vi "Init Bfr Rx - Create Buffer Options.vi"(8 "error in (no error)":errorcluster, 11 "Rx Loop Data in":T1 {"Buffer Resources"."Data Buffer" format="%016x"; "Buffer Option Support"."Ping Pong Buffer"."Active Buffer Ref" format="%016x"; "Buffer Option Support"."Cached Buffer"."Cache Buffer" format="%016x"}) -> (0 "error out":errorcluster, 3 "Rx Loop Data out":T1 {"Buffer Resources"."Data Buffer" format="%016x"; "Buffer Option Support"."Ping Pong Buffer"."Active Buffer Ref" format="%016x"; "Buffer Option Support"."Cached Buffer"."Cache Buffer" format="%016x"})   [LabVIEW 2019, in "UDP-Custom-Device Engine.lvlib"]
uses:
  UDP-Custom-Device Engine.lvlib
  Types/Engine - Buffered Rx Loop Data.ctl
  Types/Engine - General Resources.ctl
  <vilib>/NI VeriStand/VeriStand Data/Typedefs/Typedefs.Data Types.ctl
  Shared/Types/Shared - Duplex Settings.ctl
  Shared/Types/Shared - Header Details.ctl
  Types/Engine - Buffer Resources.ctl
  Shared/Types/Shared - Pointer Encoding.ctl
  Types/Engine - Rx Runtime Resources.ctl
  Types/Engine - Execution Config.ctl
  Shared/Types/Shared - Thread Management.ctl
  Types/Engine - Rx New Data Options Support.ctl
  Shared/Types/Shared - New Data Options.ctl
  Types/Engine - Buffered Rx Buffer Option Support.ctl
  Shared/Types/Shared - Receive Buffer Options.ctl
  Types/Engine - Buffered Rx Circular Buffer.ctl
  Types/Engine - Buffered Rx Cached Buffer.ctl
  Types/Engine - Buffered Rx Ping Pong Buffer.ctl
  Types/Engine - Buffered Rx Active Buffer.ctl
  Types/Engine - Buffered Rx Channel Refs.ctl
  <vilib>/NI/NIVS Inline Async API/_Data Access Engine/Data Access Engine/Types/Write.DVR.ctl
  <vilib>/NI/NIVS Inline Async API/_Data Access Engine/Access Type Classes/Write/Write.lvclass
  <vilib>/NI/NIVS Inline Async API/_Data Access Engine/Data Access Engine/Types/Read.DVR.ctl
  <vilib>/NI/NIVS Inline Async API/_Data Access Engine/Access Type Classes/Read/Read.lvclass
  Types/Engine - Buffered Rx Ping Pong Channels.ctl
  Types/Engine - Debug Resources.ctl
  <vilib>/NI/NIVS Inline Async API/_Data Access Engine/Access Type Classes/Write/Write.lvclass/Write.ctl
  <vilib>/NI VeriStand/VeriStand Data/Pointer Operations/Pointer.Write (1D U8).vi
  <vilib>/NI VeriStand/VeriStand Data/Pointer Operations/Pointer.Write (U8).vi
  <vilib>/NI VeriStand/VeriStand Data/Pointer Operations/Pointer.Write (U16).vi
  <vilib>/NI/NIVS Inline Async API/_Data Access Engine/Data Access Engine/Methods/Write.Data.vi
  <vilib>/NI/NIVS Inline Async API/_Data Access Engine/Access Type Classes/Write/Write.ProcessData.vi
  <vilib>/NI VeriStand/VeriStand Data/VeriStand Data.lvlib
  <vilib>/NI/NIVS Inline Async API/_Data Access Engine/Data Access Engine/Data Access Engine.lvclass
  Shared/UDP-Custom-Device Shared.lvlib
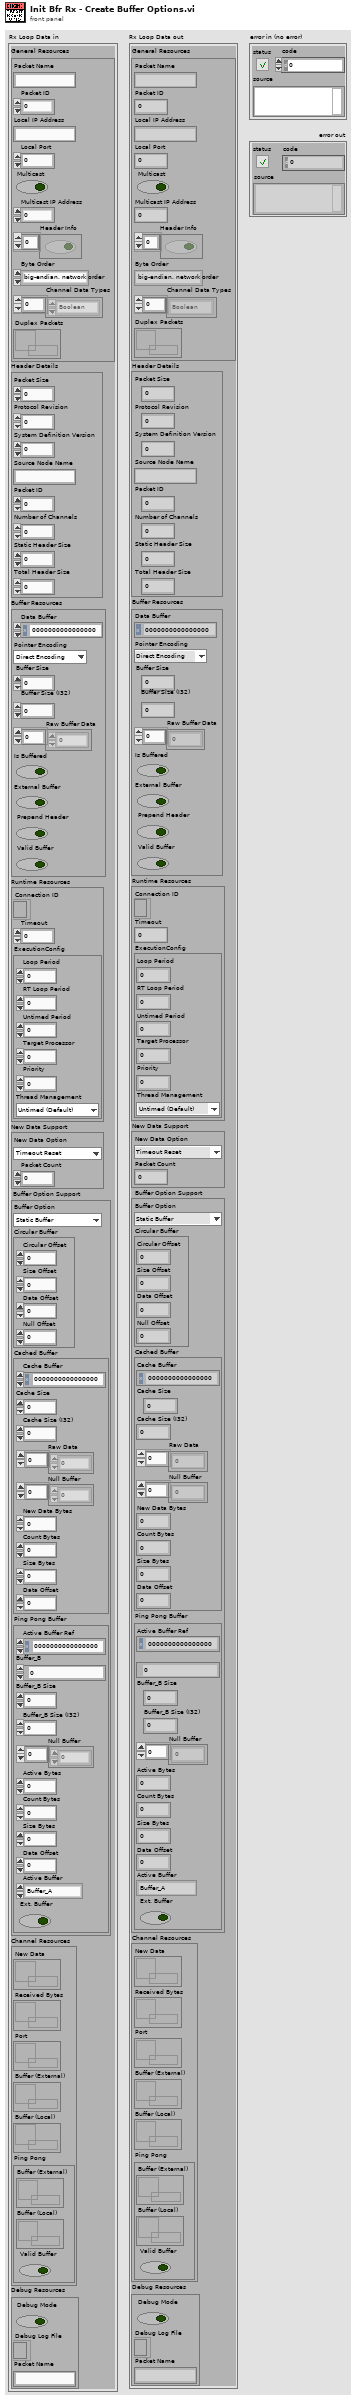
[diagram p1: front panel]
types:
  T1 = typedef "UDP-Custom-Device Engine.lvlib/Engine - Buffered Rx Loop Data.ctl" = cluster{"General Resources":T2, "Header Details":T4, "Buffer Resources":T5, "Runtime Resources":T7, "New Data Support":T10, "Buffer Option Support":T12, "Channel Resources":T18, "Debug Resources":T22}
  T2 = typedef "UDP-Custom-Device Engine.lvlib/Engine - General Resources.ctl" = cluster{"Packet Name":string, "Packet ID":i32, "Local IP Address":string, "Local Port":i32, "Multicast":bool, "Multicast IP Address":u32, "Header Info":bool[], "Byte Order":enum16{"big-endian, network order", "native, host order", "little-endian"}, "Channel Data Types":T3[], "Duplex Packets":refnum<data-value>}
  T3 = typedef "VeriStand Data.lvlib/Typedefs.Data Types.ctl" = enum16{"Boolean", "Single", "Double", "I8", "I16", "I32", "I64", "U8", "U16", "U32", "U64"}
  T4 = typedef "UDP-Custom-Device Shared.lvlib/Shared - Header Details.ctl" = cluster{"Packet Size":u16, "Protocol Revision":u8, "System Definition Version":u64, "Source Node Name":string, "Packet ID":u32, "Number of Channels":u32, "Static Header Size":u16, "Total Header Size":u16}
  T5 = typedef "UDP-Custom-Device Engine.lvlib/Engine - Buffer Resources.ctl" = cluster{"Data Buffer":u64, "Pointer Encoding":T6, "Buffer Size":u64, "Buffer Size (I32)":i32, "Raw Buffer Data":u8[], "Is Buffered":bool, "External Buffer":bool, "Prepend Header":bool, "Valid Buffer":bool}
  T6 = typedef "UDP-Custom-Device Shared.lvlib/Shared - Pointer Encoding.ctl" = enum16{"Direct Encoding", "Conversion Encoding"}
  T7 = typedef "UDP-Custom-Device Engine.lvlib/Engine - Rx Runtime Resources.ctl" = cluster{"Connection ID":refnum<k16>, "Timeout":i32, "ExecutionConfig":T8}
  T8 = typedef "UDP-Custom-Device Engine.lvlib/Engine - Execution Config.ctl" = cluster{"Loop Period":i64, "RT Loop Period":i64, "Untimed Period":u32, "Target Processor":i32, "Priority":i32, "Thread Management":T9}
  T9 = typedef "UDP-Custom-Device Shared.lvlib/Shared - Thread Management.ctl" = enum16{"Untimed (Default)", "Timed (High Priority)"}
  T10 = typedef "UDP-Custom-Device Engine.lvlib/Engine - Rx New Data Options Support.ctl" = cluster{"New Data Option":T11, "Packet Count":dbl}
  T11 = typedef "UDP-Custom-Device Shared.lvlib/Shared - New Data Options.ctl" = enum16{"Timeout Reset", "Counter"}
  T12 = typedef "UDP-Custom-Device Engine.lvlib/Engine - Buffered Rx Buffer Option Support.ctl" = cluster{"Buffer Option":T13, "Circular Buffer":T14, "Cached Buffer":T15, "Ping Pong Buffer":T16}
  T13 = typedef "UDP-Custom-Device Shared.lvlib/Shared - Receive Buffer Options.ctl" = enum16{"Static Buffer", "Circular Buffer", "Circular Buffer + Size", "Internal Cache", "Internal Cache + Size", "Ping Pong", "Ping Pong + Size"}
  T14 = typedef "UDP-Custom-Device Engine.lvlib/Engine - Buffered Rx Circular Buffer.ctl" = cluster{"Circular Offset":u64, "Size Offset":u64, "Data Offset":u64, "Null Offset":u64}
  T15 = typedef "UDP-Custom-Device Engine.lvlib/Engine - Buffered Rx Cached Buffer.ctl" = cluster{"Cache Buffer":u64, "Cache Size":u64, "Cache Size (I32)":i32, "Raw Data":u8[], "Null Buffer":u8[], "New Data Bytes":u64, "Count Bytes":u64, "Size Bytes":u64, "Data Offset":u64}
  T16 = typedef "UDP-Custom-Device Engine.lvlib/Engine - Buffered Rx Ping Pong Buffer.ctl" = cluster{"Active Buffer Ref":u64, "Buffer_B":u64, "Buffer_B Size":u64, "Buffer_B Size (I32)":i32, "Null Buffer":u8[], "Active Bytes":u64, "Count Bytes":u64, "Size Bytes":u64, "Data Offset":u64, "Active Buffer":T17, "Ext. Buffer":bool}
  T17 = typedef "UDP-Custom-Device Engine.lvlib/Engine - Buffered Rx Active Buffer.ctl" = enum16{"Buffer_A", "Buffer_B"}
  T18 = typedef "UDP-Custom-Device Engine.lvlib/Engine - Buffered Rx Channel Refs.ctl" = cluster{"New Data":T19, "Received Bytes":T19, "Port":T19, "Buffer (External)":T20, "Buffer (Local)":T19, "Ping Pong":T21}
  T19 = typedef "Data Access Engine.lvlib/Data Access Engine.lvclass/Write.DVR.ctl" = refnum<data-value>
  T20 = typedef "Data Access Engine.lvlib/Data Access Engine.lvclass/Read.DVR.ctl" = refnum<data-value>
  T21 = typedef "UDP-Custom-Device Engine.lvlib/Engine - Buffered Rx Ping Pong Channels.ctl" = cluster{"Buffer (External)":T20, "Buffer (Local)":T19, "Valid Buffer":bool}
  T22 = typedef "UDP-Custom-Device Engine.lvlib/Engine - Debug Resources.ctl" = cluster{"Debug Mode":bool, "Debug Log File":refnum<file>, "Packet Name":string}
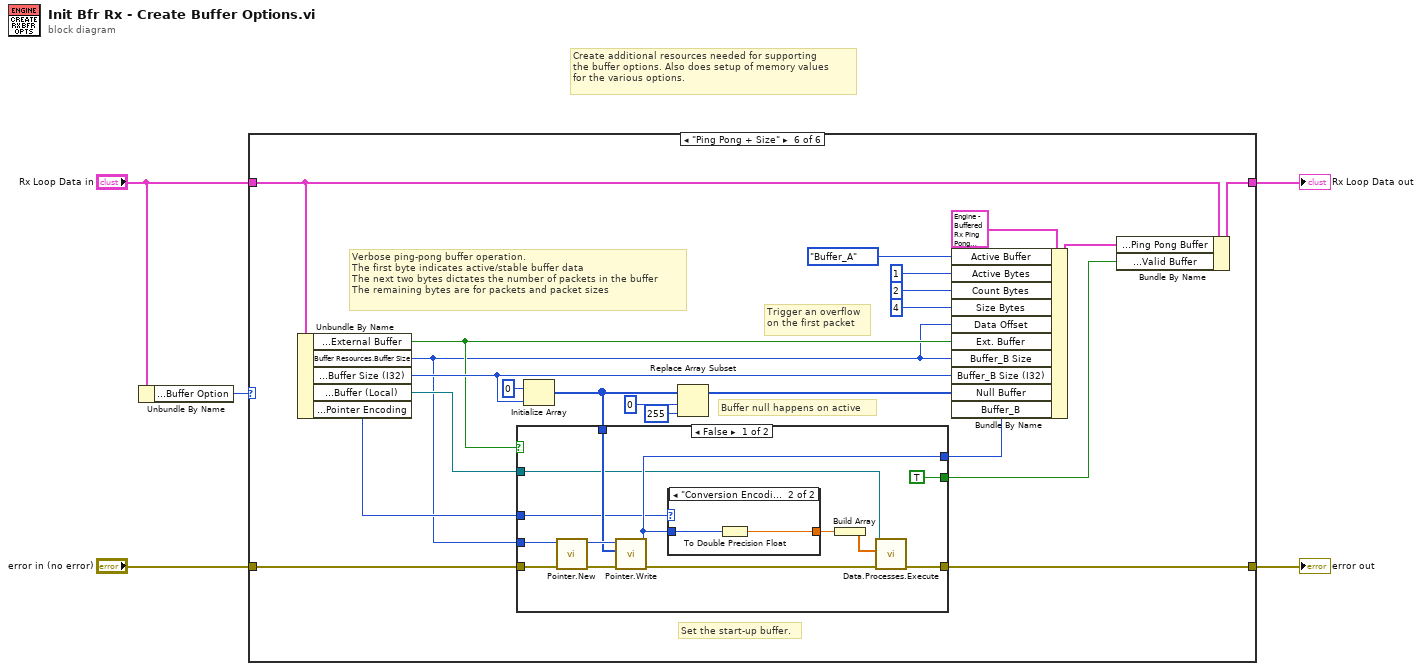
[diagram p0: block diagram]
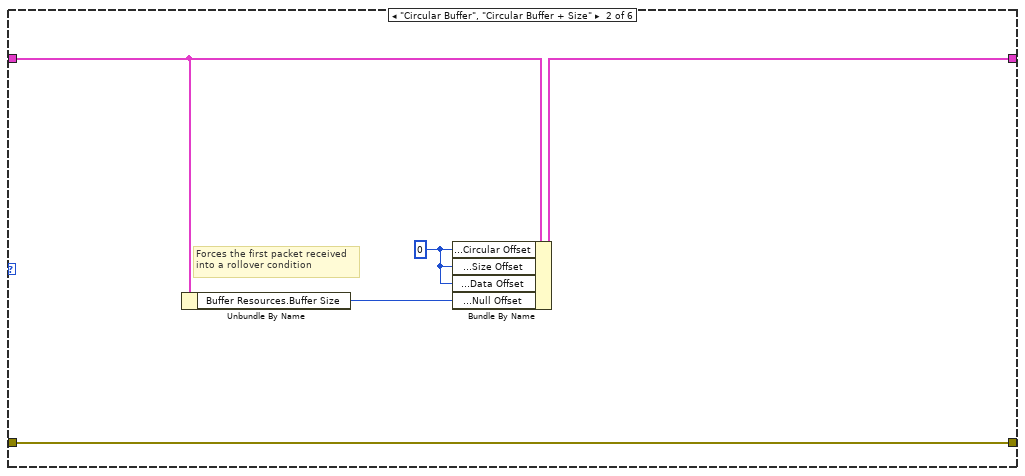
[diagram p3: hidden frame]
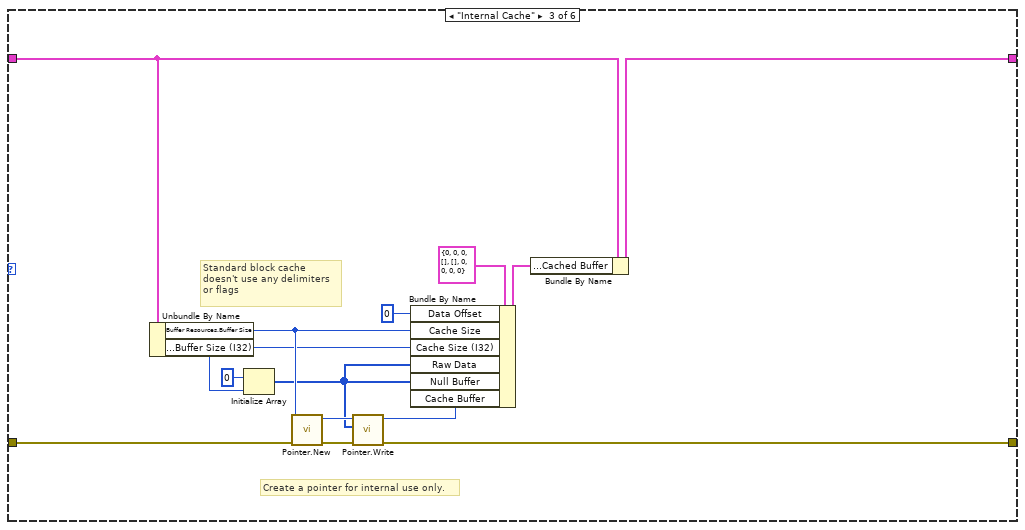
[diagram p4: hidden frame]
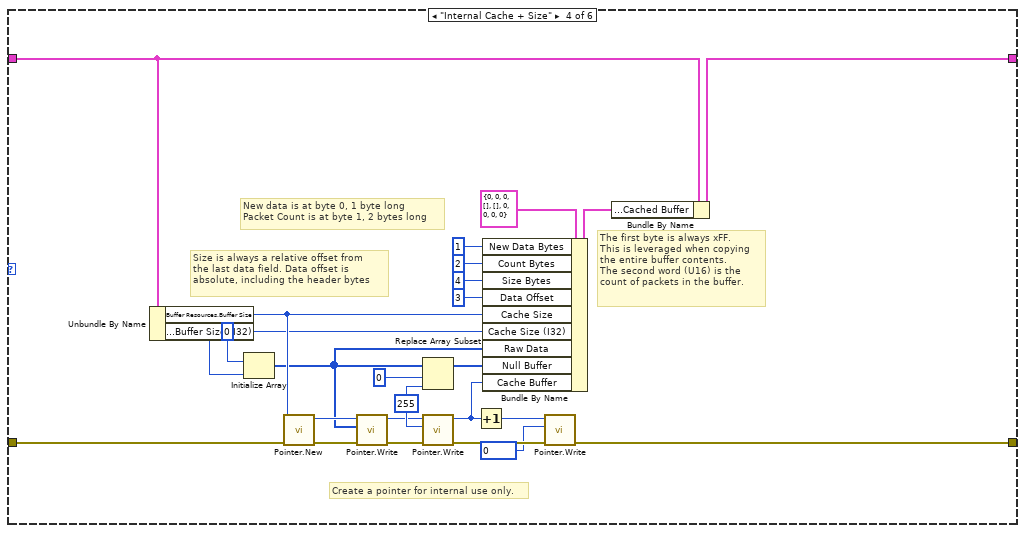
[diagram p5: hidden frame]
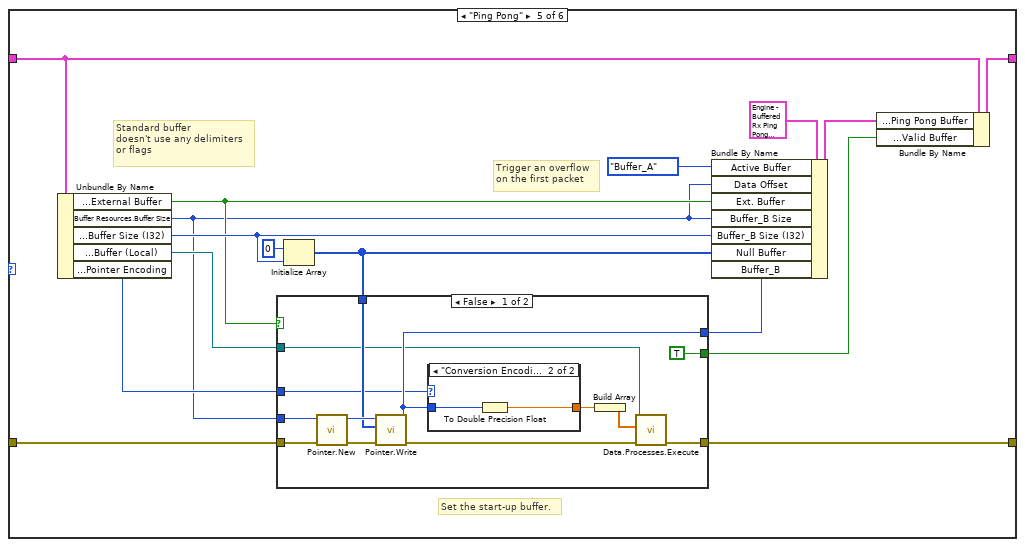
[diagram p6: hidden frame]
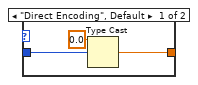
[diagram p7: hidden frame]
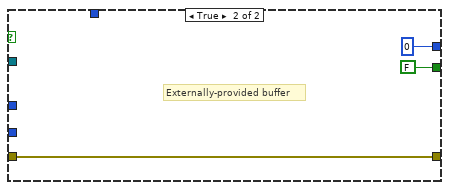
[diagram p8: hidden frame]
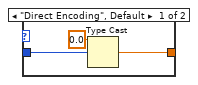
[diagram p9: hidden frame]
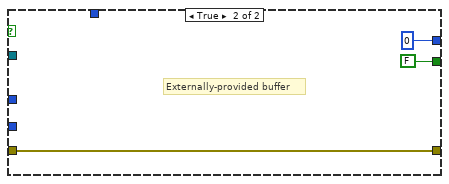
[diagram p10: hidden frame]
diagram:
  # "Create additional resources needed for supporting\nthe buffer options. Also does setup of memory values\nfor the various options."
  n1 = Unbundle By Name("Rx Loop Data in") -> ("Buffer Option Support.Buffer Option"=w1:T13)
  n2 = case shown="\"Ping Pong + Size\"" w1 {
    tunnel: [w7 w11 w26 w51 w67 w110] -> w5
    tunnel: "Rx Loop Data in" -> [w7 w10 w23 w48 w64 w107]
    tunnel: [w6 w12 w15 w38 w60 w103] -> w3
    tunnel: "error in (no error)" -> [w6 w12 w21 w45 w61 w104]
    frame Default {
    }
    frame "Circular Buffer", "Circular Buffer + Size" {
      w9 = u64 0 ("Buffer Option Support.Circular Buffer.Circular Offset")
      # "Forces the first packet received\ninto a rollover condition"
      n3 = Unbundle By Name(w10) -> ("Buffer Resources.Buffer Size"=w8:u64)
      n4 = Bundle By Name(cluster=w10, "Buffer Option Support.Circular Buffer.Circular Offset"=w9, "Buffer Option Support.Circular Buffer.Size Offset"=w9, "Buffer Option Support.Circular Buffer.Data Offset"=w9, "Buffer Option Support.Circular Buffer.Null Offset"=w8) -> (w11:T1)
    }
    frame "Internal Cache" {
      # "Standard block cache\ndoesn't use any delimiters\nor flags"
      # "Create a pointer for internal use only."
      n5 = Unbundle By Name(w23) -> ("Buffer Resources.Buffer Size"=w22:u64, "Buffer Resources.Buffer Size (I32)"=w20:i32)
      n6 = Initialize Array(u8 0 ("element"), w20) -> (w13:u8[])
      n7 = call <vilib>:"Pointer.New.vi"("error in (no error)"=w21, "size in bytes"=w22) -> ("error out"=w16:errorcluster, "pointer"=w18:u64)  [unwired: 8 in]
      n8 = call-poly <vilib>:"Pointer.Write.vi"("error in (no error)"=w16, "values"=w13, "pointer in"=w18) -> ("error out"=w15:errorcluster, "pointer out"=w17:u64)  [unwired: 6 in, 1 out]
      n9 = Bundle By Name(cluster=T15 {"Cache Buffer"=0, "Cache Size"=0, "Cache Size (I32)"=0, "Raw Data"=[], "Null Buffer"=[], "New Data Bytes"=0, "Count Bytes"=0, "Size Bytes"=0, "Data Offset"=0} ("Buffer Option Support.Cached Buffer"), "Data Offset"=u64 0 ("Buffer Option Support.Circular Buffer.Circular Offset"), "Cache Size"=w22, "Cache Size (I32)"=w20, "Raw Data"=w13, "Null Buffer"=w13, "Cache Buffer"=w17) -> (w24:T15)
      n10 = Bundle By Name(cluster=w23, "Buffer Option Support.Cached Buffer"=w24) -> (w26:T1)
    }
    frame "Internal Cache + Size" {
      w33 = u8 255 ("value")
      # "Size is always a relative offset from\nthe last data field. Data offset is\nabsolute, including the header bytes"
      # "The first byte is always xFF.\nThis is leveraged when copying\nthe entire buffer contents.\nThe second word (U16) is the\ncount of packets in the buffer."
      # "New data is at byte 0, 1 byte long\nPacket Count is at byte 1, 2 bytes long"
      # "Create a pointer for internal use only."
      n11 = Unbundle By Name(w48) -> ("Buffer Resources.Buffer Size"=w46:u64, "Buffer Resources.Buffer Size (I32)"=w44:i32)
      n12 = Initialize Array(u8 0 ("element"), w44) -> (w27:u8[])
      n13 = call <vilib>:"Pointer.New.vi"("error in (no error)"=w45, "size in bytes"=w46) -> ("error out"=w29:errorcluster, "pointer"=w31:u64)  [unwired: 8 in]
      n14 = call-poly <vilib>:"Pointer.Write.vi"("error in (no error)"=w29, "values"=w27, "pointer in"=w31) -> ("error out"=w28:errorcluster, "pointer out"=w30:u64)  [unwired: 6 in, 1 out]
      n15 = Replace Array Subset(array=w27, new element=w33, index=0) -> (w34:u8[])
      n16 = call-poly <vilib>:"Pointer.Write.vi"("error in (no error)"=w28, "value"=w33, "pointer in"=w30) -> ("error out"=w39:errorcluster, "pointer out"=w41:u64)  [unwired: 6 in, 1 out]
      n17 = Increment(x=w41) -> (x+1=w40:u64)
      n18 = Bundle By Name(cluster=T15 {"Cache Buffer"=0, "Cache Size"=0, "Cache Size (I32)"=0, "Raw Data"=[], "Null Buffer"=[], "New Data Bytes"=0, "Count Bytes"=0, "Size Bytes"=0, "Data Offset"=0} ("Buffer Option Support.Cached Buffer"), "New Data Bytes"=u64 1 ("Buffer Option Support.Circular Buffer.Circular Offset"), "Count Bytes"=u64 2 ("New Data Offset"), "Size Bytes"=u64 4 ("Buffer Option Support.Circular Buffer.Circular Offset"), "Data Offset"=u64 3, "Cache Size"=w46, "Cache Size (I32)"=w44, "Raw Data"=w27, "Null Buffer"=w34, "Cache Buffer"=w41) -> (w49:T15)
      n19 = call-poly <vilib>:"Pointer.Write.vi"("error in (no error)"=w39, "value"=u16 0, "pointer in"=w40) -> ("error out"=w38:errorcluster)  [unwired: 6 in, 2 out]
      n20 = Bundle By Name(cluster=w48, "Buffer Option Support.Cached Buffer"=w49) -> (w51:T1)
    }
    frame "Ping Pong" {
      # "Trigger an overflow\non the first packet"
      # "Set the start-up buffer."
      # "Standard buffer\ndoesn't use any delimiters\nor flags"
      n21 = Unbundle By Name(w64) -> ("Buffer Resources.External Buffer"=w59:bool, "Buffer Resources.Buffer Size"=w53:u64, "Buffer Resources.Buffer Size (I32)"=w66:i32, "Channel Resources.Ping Pong.Buffer (Local)"=w56:T19, "Buffer Resources.Pointer Encoding"=w57:T6)
      n22 = Initialize Array(u8 0 ("element"), w66) -> (w52:u8[])
      n23 = case shown="False" w59 {
        tunnel: w53 -> [w78 _]
        tunnel: w61 -> [w77 w88]
        tunnel: [w71 w88] -> w60
        tunnel: w52 -> [w76 _]
        tunnel: [w75 u64 0 ("pointer out")] -> w58
        tunnel: w57 -> [w74 _]
        tunnel: w56 -> [w70 _]
        tunnel: [TRUE FALSE] -> w55
        frame False {
          n24 = call <vilib>:"Pointer.New.vi"("error in (no error)"=w77, "size in bytes"=w78) -> ("error out"=w80:errorcluster, "pointer"=w79:u64)  [unwired: 8 in]
          n25 = call-poly <vilib>:"Pointer.Write.vi"("error in (no error)"=w80, "values"=w76, "pointer in"=w79) -> ("error out"=w72:errorcluster, "pointer out"=w75:u64)  [unwired: 6 in, 1 out]
          n26 = case shown="\"Conversion Encoding\"" w74 {
            tunnel: w75 -> [w83 w85]
            tunnel: [w82 w84] -> w73
            frame "Direct Encoding", Default {
              n27 = Type Cast(type=0.0, x=w83) -> (*(type *) &x=w82:dbl)
            }
            frame "Conversion Encoding" {
              n28 = To Double Precision Float(number=w85) -> (double precision float=w84:dbl)
            }
          }
          n29 = Build Array(w73) -> (w69:dbl[])
          n30 = call-poly <vilib>:"Data.Processes.Execute.vi"("error in (no error)"=w72, "Values"=w69, "Ref"=w70) -> ("error out"=w71:errorcluster)  [unwired: 8 in]
        }
        frame True {
          # "Externally-provided buffer"
        }
      }
      n31 = Bundle By Name(cluster=T16 {"Active Buffer Ref"=0, "Buffer_B"=0, "Buffer_B Size"=0, "Buffer_B Size (I32)"=0, "Null Buffer"=[], "Active Bytes"=0, "Count Bytes"=0, "Size Bytes"=0, "Data Offset"=0, "Active Buffer"=enum."Buffer_A", "Ext. Buffer"=FALSE} ("Ping Pong Buffer"), "Active Buffer"=Engine_-_Buffered_Rx_Active_Buffer."Buffer_A", "Data Offset"=w53, "Ext. Buffer"=w59, "Buffer_B Size"=w53, "Buffer_B Size (I32)"=w66, "Null Buffer"=w52, "Buffer_B"=w58) -> (w62:T16)
      n32 = Bundle By Name(cluster=w64, "Buffer Option Support.Ping Pong Buffer"=w62, "Channel Resources.Ping Pong.Valid Buffer"=w55) -> (w67:T1)
    }
    frame "Ping Pong + Size" {
      # "Buffer null happens on active"
      # "Trigger an overflow\non the first packet"
      # "Verbose ping-pong buffer operation.\nThe first byte indicates active/stable buffer data\nThe next two bytes dictates the number of packets in the buffer\nThe remaining bytes are for packets and packet sizes"
      # "Set the start-up buffer."
      n33 = Unbundle By Name(w107) -> ("Buffer Resources.External Buffer"=w102:bool, "Buffer Resources.Buffer Size"=w93:u64, "Buffer Resources.Buffer Size (I32)"=w109:i32, "Channel Resources.Ping Pong.Buffer (Local)"=w99:T19, "Buffer Resources.Pointer Encoding"=w100:T6)
      n34 = Initialize Array(u8 0 ("element"), w109) -> (w90:u8[])
      n35 = case shown="False" w102 {
        tunnel: w93 -> [w121 _]
        tunnel: w104 -> [w120 w131]
        tunnel: [w114 w131] -> w103
        tunnel: w90 -> [w119 _]
        tunnel: [w118 u64 0 ("pointer out")] -> w101
        tunnel: w100 -> [w117 _]
        tunnel: w99 -> [w113 _]
        tunnel: [TRUE FALSE] -> w98
        frame False {
          n36 = call <vilib>:"Pointer.New.vi"("error in (no error)"=w120, "size in bytes"=w121) -> ("error out"=w123:errorcluster, "pointer"=w122:u64)  [unwired: 8 in]
          n37 = call-poly <vilib>:"Pointer.Write.vi"("error in (no error)"=w123, "values"=w119, "pointer in"=w122) -> ("error out"=w115:errorcluster, "pointer out"=w118:u64)  [unwired: 6 in, 1 out]
          n38 = case shown="\"Conversion Encoding\"" w117 {
            tunnel: w118 -> [w126 w128]
            tunnel: [w125 w127] -> w116
            frame "Direct Encoding", Default {
              n39 = Type Cast(type=0.0, x=w126) -> (*(type *) &x=w125:dbl)
            }
            frame "Conversion Encoding" {
              n40 = To Double Precision Float(number=w128) -> (double precision float=w127:dbl)
            }
          }
          n41 = Build Array(w116) -> (w112:dbl[])
          n42 = call-poly <vilib>:"Data.Processes.Execute.vi"("error in (no error)"=w115, "Values"=w112, "Ref"=w113) -> ("error out"=w114:errorcluster)  [unwired: 8 in]
        }
        frame True {
          # "Externally-provided buffer"
        }
      }
      n43 = Replace Array Subset(array=w90, new element=u8 255 ("new element/subarray"), index=0) -> (w89:u8[])
      n44 = Bundle By Name(cluster=T16 {"Active Buffer Ref"=0, "Buffer_B"=0, "Buffer_B Size"=0, "Buffer_B Size (I32)"=0, "Null Buffer"=[], "Active Bytes"=0, "Count Bytes"=0, "Size Bytes"=0, "Data Offset"=0, "Active Buffer"=enum."Buffer_A", "Ext. Buffer"=FALSE} ("Ping Pong Buffer"), "Active Buffer"=Engine_-_Buffered_Rx_Active_Buffer."Buffer_A", "Active Bytes"=u64 1 ("New Data Bytes"), "Count Bytes"=u64 2, "Size Bytes"=u64 4, "Data Offset"=w93, "Ext. Buffer"=w102, "Buffer_B Size"=w93, "Buffer_B Size (I32)"=w109, "Null Buffer"=w89, "Buffer_B"=w101) -> (w105:T16)
      n45 = Bundle By Name(cluster=w107, "Buffer Option Support.Ping Pong Buffer"=w105, "Channel Resources.Ping Pong.Valid Buffer"=w98) -> (w110:T1)
    }
  }
  "Rx Loop Data out" <- w5
  "error out" <- w3
